vi "NMEA_GPGGA_ToStringArray.vi"(9 "Error In":errorcluster, 10 "$GPGGA-message_IN":T2={"TimeStamp"=timestamp(0 s since 1904-01-01), "Latitude"=0.0, "Latitude-Direction"=enum."", "Longitude"=1.0, "Longitude-Direction"=enum."", "GPS-Quality"=enum."GPS fix (SPS)", "Number of Satellites"=0, "Horizontal Dilution of Precision"=0.0, "Altitude above Mean-Sea-Level"=0.0, "Geoidal separation"=0.0, "Time since last DGPS update"=0.0, "DGPS reference station ID"=0} {"Time since last DGPS update" format="%.02f [s]"; "Geoidal separation" format="%.02f [m]"; "Altitude above Mean-Sea-Level" format="%.02f [m]"; "Horizontal Dilution of Precision" format="%.02f [HDOP]"; "Longitude" format="%0.4f [long]"; "Latitude" format="%.04f [lat]"; "TimeStamp" format="%<%.2X>T"}) -> (1 "Error Out":errorcluster, 2 "$GPGGA-message_OUT":string[](array[string]))   [LabVIEW 2016, in "AIRMAR WeatherCaster.lvlib"]
doc: "<B>GPGGA</B>\nGlobal Positioning System Fix Data"
uses:
  AIRMAR WeatherCaster.lvlib
  NMEA_GPGGA-data.ctl
  NMEA_LatitudeDirection.ctl
  NMEA_LongitudeDirection.ctl
  NMEA_GPS-Quality.ctl
panel:
  out "GPS-Quality":T1
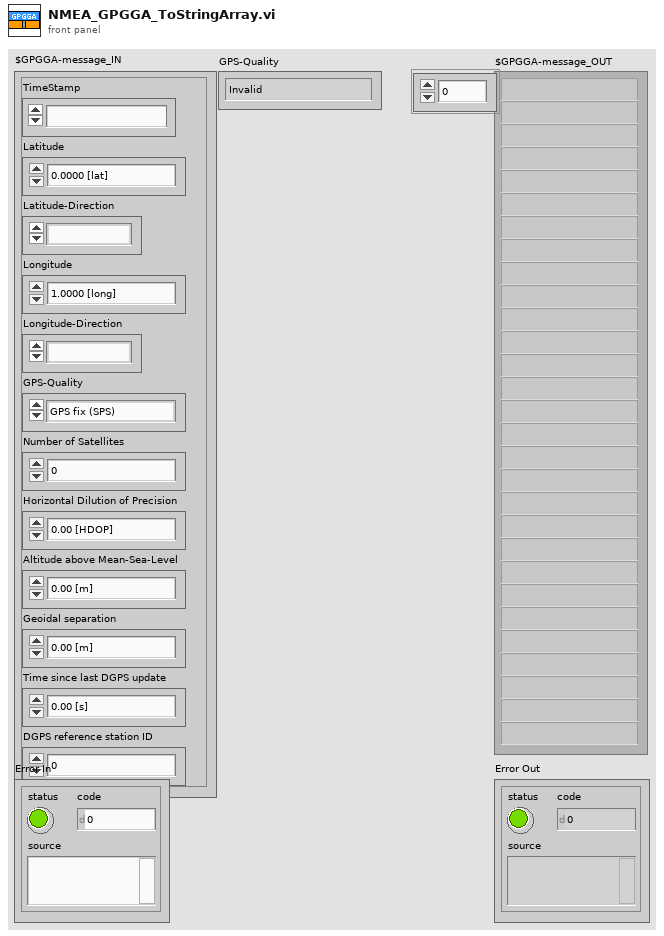
[diagram p1: front panel]
types:
  T1 = typedef "AIRMAR WeatherCaster.lvlib/NMEA_GPS-Quality.ctl" = enum16{"Invalid", "GPS fix (SPS)", "DGPS fix", "PPS fix", "Real Time Kinematic", "Float RTK", "estimated", "Manual input mode", "Simulation mode"}
  T2 = typedef "AIRMAR WeatherCaster.lvlib/NMEA_GPGGA-data.ctl" = cluster{"TimeStamp":timestamp, "Latitude":dbl, "Latitude-Direction":T3, "Longitude":dbl, "Longitude-Direction":T4, "GPS-Quality":T1, "Number of Satellites":i32, "Horizontal Dilution of Precision":dbl, "Altitude above Mean-Sea-Level":dbl, "Geoidal separation":dbl, "Time since last DGPS update":dbl, "DGPS reference station ID":i32}
  T3 = typedef "AIRMAR WeatherCaster.lvlib/NMEA_LatitudeDirection.ctl" = enum16{"", "North", "South"}
  T4 = typedef "AIRMAR WeatherCaster.lvlib/NMEA_LongitudeDirection.ctl" = enum16{"", "East", "West"}
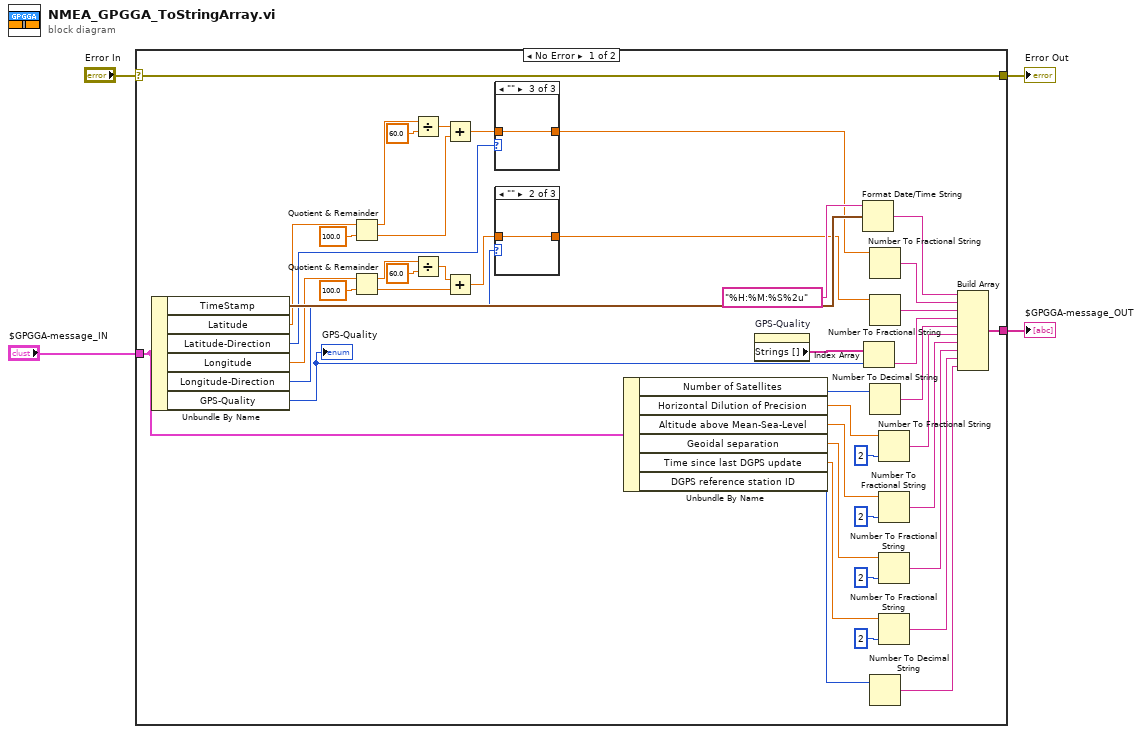
[diagram p0: block diagram]
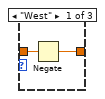
[diagram p2: hidden frame]
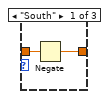
[diagram p4: hidden frame]
diagram:
  n1 = case shown="No Error" "Error In" {
    selector: "Error In" -> [w49 w58]
    tunnel: "$GPGGA-message_IN" -> [w44 _]
    tunnel: [w49 w58] -> w4
    tunnel: [w27 _] -> w1
    frame No Error {
      n2 = Unbundle By Name(w44) -> ("TimeStamp"=w48:timestamp, "Latitude"=w9:dbl, "Latitude-Direction"=w10:T3, "Longitude"=w7:dbl, "Longitude-Direction"=w8:T4, "GPS-Quality"=w45:T1)
      "GPS-Quality" <- w45
      n3 = Quotient & Remainder(x=w9, y=100.0) -> (x-y*floor(x/y)=w11:dbl, floor(x/y)=w13:dbl)
      n4 = Quotient & Remainder(x=w7, y=100.0) -> (x-y*floor(x/y)=w20:dbl, floor(x/y)=w18:dbl)
      n5 = Divide(x=w11, y=60.0) -> (x/y=w14:dbl)
      n6 = Divide(x=w20, y=60.0) -> (x/y=w17:dbl)
      n7 = Add(x=w14, y=w13) -> (x+y=w15:dbl)
      n8 = Add(x=w17, y=w18) -> (x+y=w16:dbl)
      n9 = case shown="\"\"" w10 {
        tunnel: w15 -> [w55 w56 w57]
        tunnel: [w54 w56 w57] -> w6
        frame "South" {
          n10 = Negate(x=w55) -> (-x=w54:dbl)
        }
        frame "North" {
        }
        frame "" {
        }
      }
      n11 = case shown="\"\"" w8 {
        tunnel: w16 -> [w51 w52 w53]
        tunnel: [w50 w52 w53] -> w5
        frame "West" {
          n12 = Negate(x=w51) -> (-x=w50:dbl)
        }
        frame "" {
        }
        frame "East" {
        }
      }
      n13 = Unbundle By Name(w44) -> ("Number of Satellites"=w43:i32, "Horizontal Dilution of Precision"=w42:dbl, "Altitude above Mean-Sea-Level"=w41:dbl, "Geoidal separation"=w40:dbl, "Time since last DGPS update"=w39:dbl, "DGPS reference station ID"=w38:i32)
      n14 = property on="GPS-Quality" class="Enum (strict)"() -> ("Strings []"=w46:string[])  [unwired: 2 in, 2 out]
      n15 = Format Date/Time String(time format string (%c)="%H:%M:%S%2u" ("chaîne de format de l'heure (%c)"), seconds (now)=w48) -> (date/time string=w37:string)  [unwired: 1 in]
      n16 = Index Array(array=w46, index=w45) -> (element=w34:string)
      n17 = Number To Fractional String(number=w6) -> (F-format string=w36:string)  [unwired: 3 in]
      n18 = Number To Fractional String(number=w5) -> (F-format string=w35:string)  [unwired: 3 in]
      n19 = Number To Decimal String(number=w43) -> (decimal integer string=w33:string)  [unwired: 1 in]
      n20 = Number To Decimal String(number=w38) -> (decimal integer string=w28:string)  [unwired: 1 in]
      n21 = Number To Fractional String(number=w42, precision (6)=i16 2 ("précision (6)")) -> (F-format string=w32:string)  [unwired: 2 in]
      n22 = Number To Fractional String(number=w41, precision (6)=i16 2 ("précision (6)")) -> (F-format string=w31:string)  [unwired: 2 in]
      n23 = Number To Fractional String(number=w40, precision (6)=i16 2 ("précision (6)")) -> (F-format string=w30:string)  [unwired: 2 in]
      n24 = Number To Fractional String(number=w39, precision (6)=i16 2 ("précision (6)")) -> (F-format string=w29:string)  [unwired: 2 in]
      n25 = Build Array(w37, w36, w35, w34, w33, w32, w31, w30, w29, w28) -> (w27:string[])
    }
    frame Error {
    }
  }
  "Error Out" <- w4
  "$GPGGA-message_OUT" <- w1
